vi "Set Cooler ON - OFF.vi"(8 "error in (no error)":errorcluster, 11 "Cooler in":refnum<class "Cooler.lvclass">) -> (0 "error out":errorcluster, 3 "Cooler out":refnum<class "Cooler.lvclass">)   [LabVIEW 2018, in "Cooler.lvclass"]
uses:
  Cooler.lvclass
  C:/Users/observer/Desktop/SPARC4_ACS/SPARC4_ACS/Simulated_Cooler/Simulated_Cooler.lvclass
  Simulated_Cooler/Simulated_Cooler.lvclass
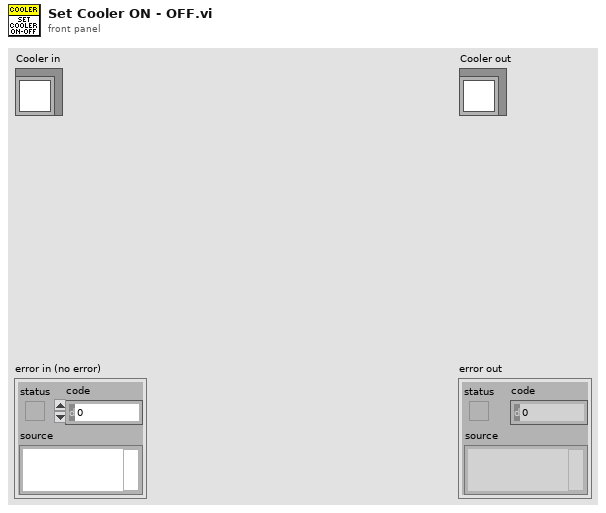
[diagram p1: front panel]
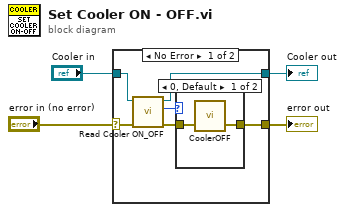
[diagram p0: block diagram]
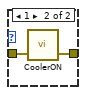
[diagram p2: hidden frame]
diagram:
  n1 = case shown="No Error" "error in (no error)" {
    selector: "error in (no error)" -> [w5 w16]
    tunnel: [w10 w16] -> w2
    tunnel: [w8 w15] -> w3
    tunnel: "Cooler in" -> [w9 w15]
    frame No Error {
      n2 = call "Read Cooler ON_OFF.vi"("error in (no error)"=w5, "Cooler in"=w9) -> ("error out"=w7:errorcluster, "Cooler ON/OFF"=w6:u8, "Cooler out"=w8:refnum<class "Cooler.lvclass">)  [unwired: 7 in]
      n3 = case shown="0, Default" w6 {
        tunnel: w7 -> [w12 w14]
        tunnel: [w11 w13] -> w10
        frame 0, Default {
          n4 = call <userlib>:"CoolerOFF.vi"("error in (no error)"=w12) -> ("error out"=w11:errorcluster)  [unwired: 1 in, 1 out]
        }
        frame 1 {
          n5 = call <userlib>:"CoolerON.vi"("error in (no error)"=w14) -> ("error out"=w13:errorcluster)  [unwired: 1 in, 1 out]
        }
      }
    }
    frame Error {
    }
  }
  "error out" <- w2
  "Cooler out" <- w3
